vi "Axis Sensitivity.vi"(10 "Raw":dbl, 11 "Sensitivity":dbl) -> (3 "Output":dbl)   [LabVIEW 2014, in "hhVI.lvlib"]
uses:
  hhVI.lvlib
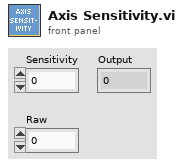
[diagram p1: front panel]
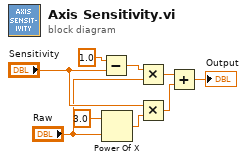
[diagram p0: block diagram]
diagram:
  n1 = Subtract(x=1.0, y="Sensitivity") -> (x-y=w5:dbl)
  n2 = Power Of X(1:"Raw", 2:3.0 ("y")) -> (0:w8:dbl)
  n3 = Multiply(x=w5, y="Raw") -> (x*y=w2:dbl)
  n4 = Multiply(x="Sensitivity", y=w8) -> (x*y=w1:dbl)
  n5 = Add(x=w2, y=w1) -> (x+y=→"Output":dbl)
